vi "MainVI.vi"() -> ()   [LabVIEW 2025]
panel:
  out "STOP OPERATION":bool
  in  "R_Manual Control":bool
  in  "R_PID Control":bool
  in  "Force VI":bool
  in  "Temp VI":bool
  in  "AI VI":bool
  in  "AO VI":bool
  # "Weber State Rocket Control"
  # "DAQ Modules Operation"
  # "Live Test Operation"
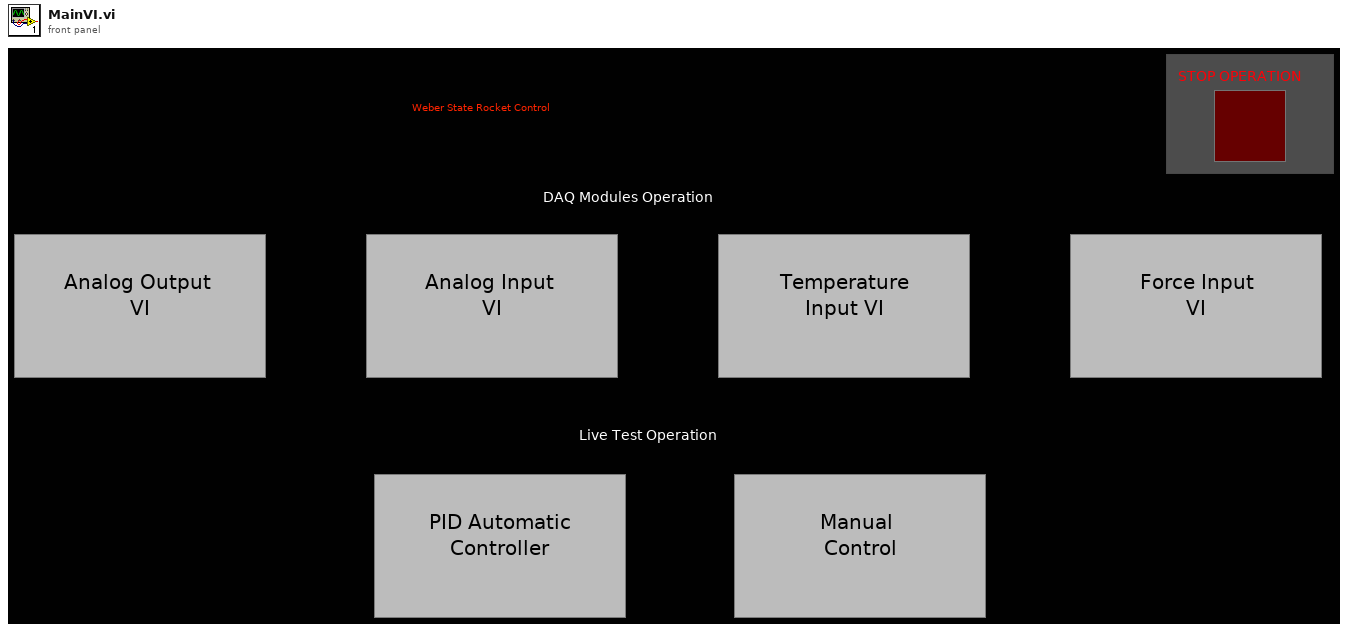
[diagram p1: front panel]
types:
  T1 = enum16{"Init", "Idle", "Run Analog Input", "Run Analog Output", "Run Temperature Input", "Rocket_Manual_Control", "Rocket_PID_Control", "Run Force Input", "Stop"}
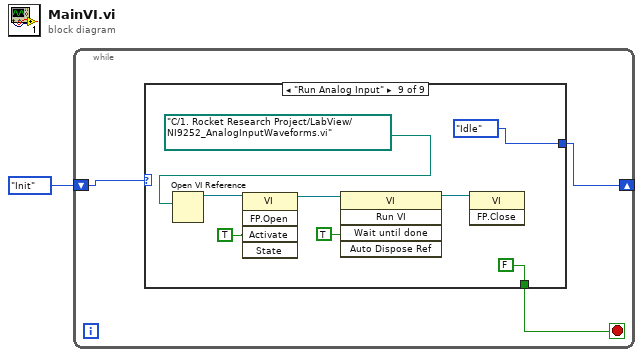
[diagram p0: block diagram]
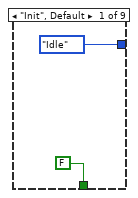
[diagram p2: hidden frame]
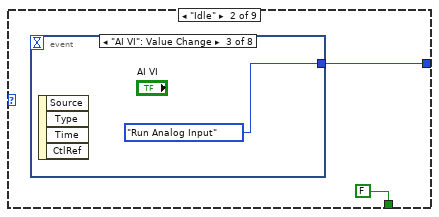
[diagram p3: hidden frame]
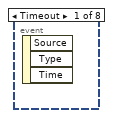
[diagram p4: hidden frame]
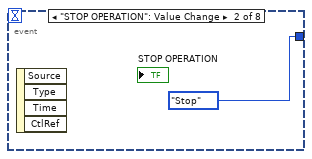
[diagram p5: hidden frame]
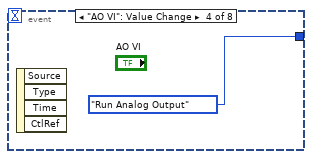
[diagram p6: hidden frame]
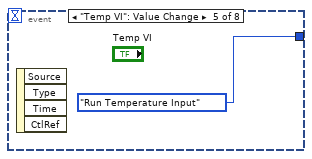
[diagram p7: hidden frame]
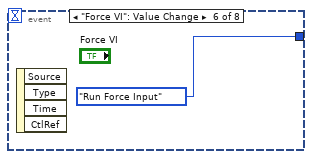
[diagram p8: hidden frame]
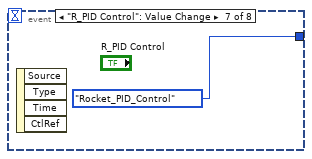
[diagram p9: hidden frame]
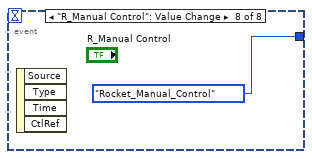
[diagram p10: hidden frame]
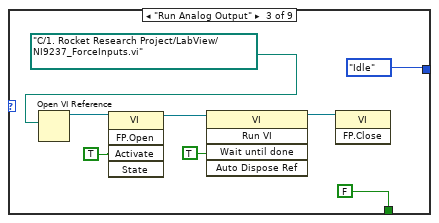
[diagram p11: hidden frame]
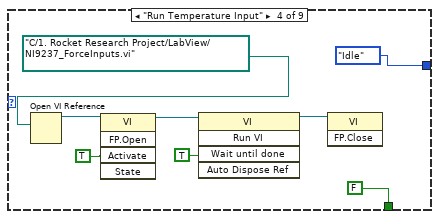
[diagram p12: hidden frame]
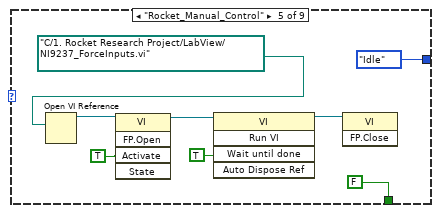
[diagram p13: hidden frame]
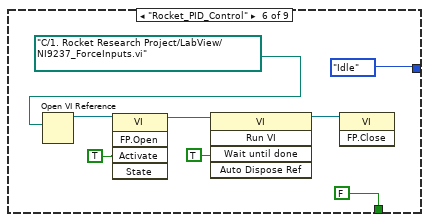
[diagram p14: hidden frame]
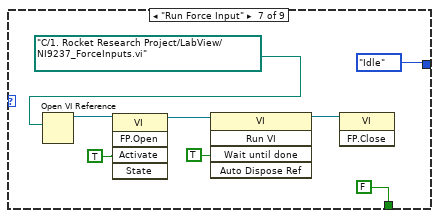
[diagram p15: hidden frame]
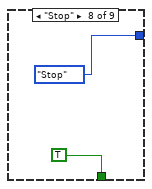
[diagram p16: hidden frame]
diagram:
  n1 = while {
    shift-right: [w3] -> _
    shift-left: T1."Init" -> [w4]
    stop <- w2 stop-if-true
    n2 = case shown="\"Run Analog Input\"" w4 {
      tunnel: [T1."Idle" w8 T1."Idle" T1."Idle" T1."Idle" T1."Idle" T1."Idle" T1."Stop" T1."Idle"] -> w3
      tunnel: [FALSE FALSE FALSE FALSE FALSE FALSE FALSE TRUE FALSE] -> w2
      frame "Init", Default {
      }
      frame "Idle" {
        n3 = event shown="[2] \"AI VI\": Value Change" {
          selector: _ -> [_ _ _ _ _ _ _ _]
          dyn-events: _ -> [_ _ _ _ _ _ _ _]
          timeout: _ -> [_ _ _ _ _ _ _ _]
          tunnel: [_ T1."Stop" T1."Run Analog Input" T1."Run Analog Output" T1."Run Temperature Input" T1."Run Force Input" T1."Rocket_PID_Control" T1."Rocket_Manual_Control"] -> w8
          event Timeout {
            n4 = event-data() -> ()  [unwired: 1 in, 3 out]
          }
          event "STOP OPERATION": Value Change {
            n5 = event-data() -> ()  [unwired: 1 in, 4 out]
          }
          event "AI VI": Value Change {
            n6 = event-data() -> ()  [unwired: 1 in, 4 out]
          }
          event "AO VI": Value Change {
            n7 = event-data() -> ()  [unwired: 1 in, 4 out]
          }
          event "Temp VI": Value Change {
            n8 = event-data() -> ()  [unwired: 1 in, 4 out]
          }
          event "Force VI": Value Change {
            n9 = event-data() -> ()  [unwired: 1 in, 4 out]
          }
          event "R_PID Control": Value Change {
            n10 = event-data() -> ()  [unwired: 1 in, 4 out]
          }
          event "R_Manual Control": Value Change {
            n11 = event-data() -> ()  [unwired: 1 in, 4 out]
          }
        }
      }
      frame "Run Analog Output" {
        n12 = Open VI Reference(vi path=path "C:/1. Rocket Research Project/LabView/NI9237_ForceInputs.vi") -> (vi reference=w20:refnum<vi>)  [unwired: 5 in, 1 out]
        n13 = invoke class="VI" method="FP.Open"(reference=w20, "Activate"=TRUE ("Activate?")) -> (reference out=w17:refnum<vi>)  [unwired: 3 in, 4 out]
        n14 = invoke class="VI" method="Run VI"(reference=w17, "Wait until done"=TRUE ("Wait Until Done")) -> (reference out=w19:refnum<vi>)  [unwired: 3 in, 4 out]
        n15 = invoke class="VI" method="FP.Close"(reference=w19) -> ()  [unwired: 2 in, 3 out]
      }
      frame "Run Temperature Input" {
        n16 = Open VI Reference(vi path=path "C:/1. Rocket Research Project/LabView/NI9237_ForceInputs.vi") -> (vi reference=w28:refnum<vi>)  [unwired: 5 in, 1 out]
        n17 = invoke class="VI" method="FP.Open"(reference=w28, "Activate"=TRUE ("Activate?")) -> (reference out=w25:refnum<vi>)  [unwired: 3 in, 4 out]
        n18 = invoke class="VI" method="Run VI"(reference=w25, "Wait until done"=TRUE ("Wait Until Done")) -> (reference out=w27:refnum<vi>)  [unwired: 3 in, 4 out]
        n19 = invoke class="VI" method="FP.Close"(reference=w27) -> ()  [unwired: 2 in, 3 out]
      }
      frame "Rocket_Manual_Control" {
        n20 = Open VI Reference(vi path=path "C:/1. Rocket Research Project/LabView/NI9237_ForceInputs.vi") -> (vi reference=w36:refnum<vi>)  [unwired: 5 in, 1 out]
        n21 = invoke class="VI" method="FP.Open"(reference=w36, "Activate"=TRUE ("Activate?")) -> (reference out=w33:refnum<vi>)  [unwired: 3 in, 4 out]
        n22 = invoke class="VI" method="Run VI"(reference=w33, "Wait until done"=TRUE ("Wait Until Done")) -> (reference out=w35:refnum<vi>)  [unwired: 3 in, 4 out]
        n23 = invoke class="VI" method="FP.Close"(reference=w35) -> ()  [unwired: 2 in, 3 out]
      }
      frame "Rocket_PID_Control" {
        n24 = Open VI Reference(vi path=path "C:/1. Rocket Research Project/LabView/NI9237_ForceInputs.vi") -> (vi reference=w44:refnum<vi>)  [unwired: 5 in, 1 out]
        n25 = invoke class="VI" method="FP.Open"(reference=w44, "Activate"=TRUE ("Activate?")) -> (reference out=w41:refnum<vi>)  [unwired: 3 in, 4 out]
        n26 = invoke class="VI" method="Run VI"(reference=w41, "Wait until done"=TRUE ("Wait Until Done")) -> (reference out=w43:refnum<vi>)  [unwired: 3 in, 4 out]
        n27 = invoke class="VI" method="FP.Close"(reference=w43) -> ()  [unwired: 2 in, 3 out]
      }
      frame "Run Force Input" {
        n28 = Open VI Reference(vi path=path "C:/1. Rocket Research Project/LabView/NI9237_ForceInputs.vi") -> (vi reference=w52:refnum<vi>)  [unwired: 5 in, 1 out]
        n29 = invoke class="VI" method="FP.Open"(reference=w52, "Activate"=TRUE ("Activate?")) -> (reference out=w49:refnum<vi>)  [unwired: 3 in, 4 out]
        n30 = invoke class="VI" method="Run VI"(reference=w49, "Wait until done"=TRUE ("Wait Until Done")) -> (reference out=w51:refnum<vi>)  [unwired: 3 in, 4 out]
        n31 = invoke class="VI" method="FP.Close"(reference=w51) -> ()  [unwired: 2 in, 3 out]
      }
      frame "Stop" {
      }
      frame "Run Analog Input" {
        n32 = Open VI Reference(vi path=path "C:/1. Rocket Research Project/LabView/NI9252_AnalogInputWaveforms.vi") -> (vi reference=w64:refnum<vi>)  [unwired: 5 in, 1 out]
        n33 = invoke class="VI" method="FP.Open"(reference=w64, "Activate"=TRUE ("Activate?")) -> (reference out=w61:refnum<vi>)  [unwired: 3 in, 4 out]
        n34 = invoke class="VI" method="Run VI"(reference=w61, "Wait until done"=TRUE ("Wait Until Done")) -> (reference out=w63:refnum<vi>)  [unwired: 3 in, 4 out]
        n35 = invoke class="VI" method="FP.Close"(reference=w63) -> ()  [unwired: 2 in, 3 out]
      }
    }
  }
